vi "Power Law Fit with Offset.vi"(6 "method (LS)":T4 items=["Least Square", "Least Absolute Residual", "Bisquare"], 7 "Poisson Weight":bool, 8 "Error In":errorcluster, 9 "tolerance (1E-4)":dbl=0.0001 format="%#_3g", 10 "Weight (none)":dbl[](array[numeric]), 11 "Plot":T3) -> (0 "Error Out":errorcluster, 1 "Power Law with Baseline Fit":T3, 2 "Power Law Fit Results":T1, 3 "Power Law Fit":T3, 4 "Power Law + Baselien Fit Results":T1)   [LabVIEW 2021, in "AlliGator Camera Noise Influence on Lifetime.lvlib"]
uses:
  AlliGator Camera Noise Influence on Lifetime.lvlib
  Graphs/XY Graph/XY Graph Plot Data.ctl
  <vilib>/Analysis/6fits.llb/Curve Fitting Criteria.ctl
  Decay Fit Parameter Map/AlliGator Power Law Fit Results.ctl
  Power Law Parameters.ctl
  <userlib>/_OpenG.lib/array/array.llb/Filter 1D Array with Scalar (DBL)__ogtk.vi
  <userlib>/_OpenG.lib/array/array.llb/Delete Elements from 1D Array (DBL)__ogtk.vi
  <vilib>/Analysis/NI_AALPro.lvlib
  Error/Error.lvlib
  <userlib>/_OpenG.lib/array/array.llb/openg_array.lvlib
  Graphs/XY Graph/XY Graph Add-Ons.lvlib
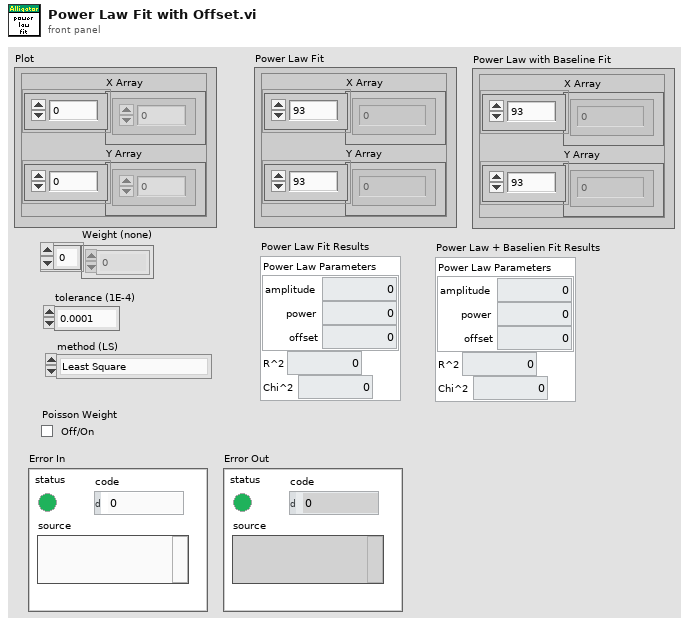
[diagram p1: front panel]
types:
  T1 = typedef "AlliGator Camera Noise Influence on Lifetime.lvlib/AlliGator Power Law Fit Results.ctl" = cluster{"Power Law Parameters":T2, "R^2":dbl, "Chi^2":dbl}
  T2 = typedef "AlliGator Camera Noise Influence on Lifetime.lvlib/Power Law Parameters.ctl" = cluster{"amplitude":dbl, "power":dbl, "offset":dbl}
  T3 = typedef "XY Graph Add-Ons.lvlib/XY Graph Plot Data.ctl" = cluster{"X Array":dbl[], "Y Array":dbl[]}
  T4 = typedef "NI_AALPro.lvlib/Curve Fitting Criteria.ctl" = u16
  T5 = cluster{"Power Law Parameters":T2, "R^2":dbl, "Chi^2":dbl}
  T6 = cluster{"amp min":dbl, "amp max":dbl, "power min":dbl, "power max":dbl, "offset min":dbl, "offset max":dbl}
  T7 = cluster{"amplitude":dbl, "power":dbl, "offset":dbl}
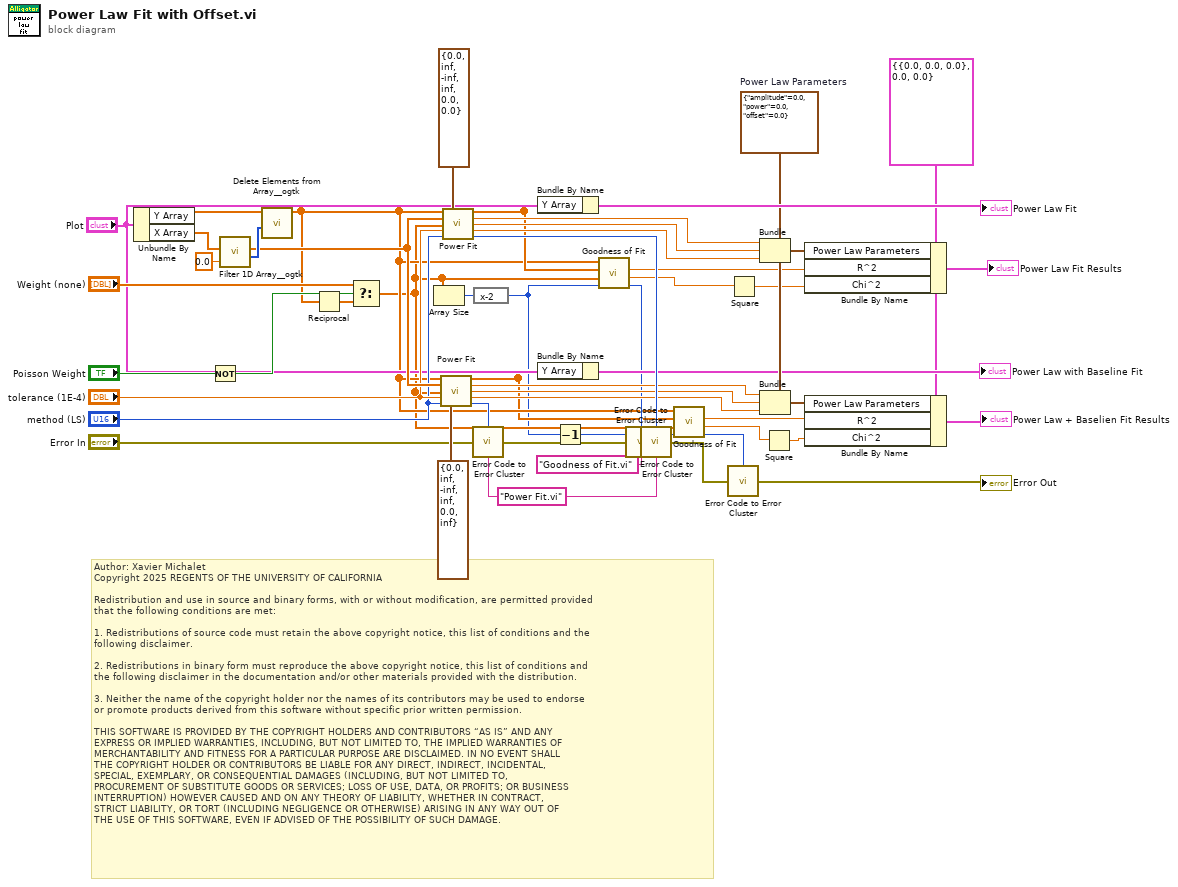
[diagram p0: block diagram]
diagram:
  w3 = T5 {"Power Law Parameters"={"amplitude"=0.0, "power"=0.0, "offset"=0.0}, "R^2"=0.0, "Chi^2"=0.0} ("Power Law + Baselien Fit Results")
  w32 = "Power Fit.vi" ("Error Source")
  w27 = T7 {"amplitude"=0.0, "power"=0.0, "offset"=0.0}  # Power Law Parameters
  # "Author: Xavier Michalet\nCopyright 2025 REGENTS OF THE UNIVERSITY OF CALIFORNIA\n\nRedistribution and use in source and binary forms, with or without modification, are permitted provided\nthat the following conditions are met:\n\n1. Redistributions of source code must retain the above copyright notice, this list of conditions and the\nfollowing disclaimer.\n\n2. Redistributions in binary form must reproduce the above copyright notice, this list of conditions and\nthe following disclaimer in the documentation and/or other materials provided with the distribution.\n\n3. Neither the name of the copyright holder nor the names of its contributors may be used to endorse \nor promote products derived from this software without specific prior written permission.\n\nTHIS SOFTWARE IS PROVIDED BY THE COPYRIGHT HOLDERS AND CONTRIBUTORS “AS IS” AND ANY \nEXPRESS OR IMPLIED WARRANTIES, INCLUDING, BUT NOT LIMITED TO, THE IMPLIED WARRANTIES OF\nMERCHANTABILITY AND FITNESS FOR A PARTICULAR PURPOSE ARE DISCLAIMED. IN NO EVENT SHALL\nTHE COPYRIGHT HOLDER OR CONTRIBUTORS BE LIABLE FOR ANY DIRECT, INDIRECT, INCIDENTAL, \nSPECIAL, EXEMPLARY, OR CONSEQUENTIAL DAMAGES (INCLUDING, BUT NOT LIMITED TO, \nPROCUREMENT OF SUBSTITUTE GOODS OR SERVICES; LOSS OF USE, DATA, OR PROFITS; OR BUSINESS\nINTERRUPTION) HOWEVER CAUSED AND ON ANY THEORY OF LIABILITY, WHETHER IN CONTRACT, \nSTRICT LIABILITY, OR TORT (INCLUDING NEGLIGENCE OR OTHERWISE) ARISING IN ANY WAY OUT OF\nTHE USE OF THIS SOFTWARE, EVEN IF ADVISED OF THE POSSIBILITY OF SUCH DAMAGE."
  n1 = Unbundle By Name("Plot") -> ("Y Array"=w47:dbl[], "X Array"=w46:dbl[])
  n2 = Not(x="Poisson Weight") -> (.not. x?=w41:bool)
  n3 = call-poly <userlib>:"Filter 1D Array__ogtk.vi"("items to filter"=0.0, "array"=w46) -> ("filtered item indices"=w44:i32[], "filtered array"=w38:dbl[])  [unwired: 4 in]
  n4 = call-poly <userlib>:"Delete Elements from Array__ogtk.vi"("indices"=w44, "array"=w47) -> ("array w/ subset deleted"=w15:dbl[])  [unwired: 8 in, 1 out]
  n5 = Reciprocal(x=w15) -> (1/x=w40:dbl[])
  n6 = Select(t="Weight (none)", s=w41, f=w40) -> (s? t:f=w13:dbl[])
  n7 = Array Size(array=w13) -> (size(s)=w24:i32)
  n8 = call <vilib>:"Power Fit.vi"("Y"=w15, "X"=w38, "Weight"=w13, "tolerance"="tolerance (1E-4)", "method"="method (LS)", "parameter bounds"=T6 {"amp min"=0.0, "amp max"=inf, "power min"=-inf, "power max"=inf, "offset min"=0.0, "offset max"=inf}) -> ("Best Power Fit"=w14:dbl[], "amplitude"=w30:dbl, "power"=w29:dbl, "offset"=w28:dbl, "error"=w34:i32)  [unwired: 4 in, 1 out]
  n9 = call <vilib>:"Power Fit.vi"("Y"=w15, "X"=w38, "Weight"=w13, "tolerance"="tolerance (1E-4)", "method"="method (LS)", "parameter bounds"=T6 {"amp min"=0.0, "amp max"=inf, "power min"=-inf, "power max"=inf, "offset min"=0.0, "offset max"=0.0}) -> ("Best Power Fit"=w25:dbl[], "amplitude"=w51:dbl, "power"=w50:dbl, "offset"=w49:dbl, "error"=w48:i32)  [unwired: 4 in, 1 out]
  n10 = call "Error Code to Error Cluster.vi"("Error Code"=w34, "Error Source"=w32, "Error In"="Error In") -> ("Error Out"=w22:errorcluster)  [unwired: 12 in]
  n11 = expression code="x-2"(w24) -> (w12:i32)
  n12 = Bundle By Name(cluster="Plot", "Y Array"=w25) -> (→"Power Law Fit":T3)
  n13 = Bundle By Name(cluster="Plot", "Y Array"=w14) -> (→"Power Law with Baseline Fit":T3)
  n14 = Decrement(x=w12) -> (x-1=w11:i32)
  n15 = call <vilib>:"Goodness of Fit.vi"("degree of freedom"=w12, "Weight"=w13, "Best Fit"=w25, "Y"=w15) -> ("error"=w23:i32, "RMSE"=w17:dbl, "R-square"=w18:dbl)  [unwired: 4 in, 1 out]
  n16 = call "Error Code to Error Cluster.vi"("Error Code"=w23, "Error Source"="Goodness of Fit.vi", "Error In"=w22) -> ("Error Out"=w21:errorcluster)  [unwired: 12 in]
  n17 = call "Error Code to Error Cluster.vi"("Error Code"=w48, "Error Source"=w32, "Error In"=w21) -> ("Error Out"=w9:errorcluster)  [unwired: 12 in]
  n18 = call <vilib>:"Goodness of Fit.vi"("degree of freedom"=w11, "Weight"=w13, "Best Fit"=w14, "Y"=w15) -> ("error"=w8:i32, "RMSE"=w5:dbl, "R-square"=w6:dbl)  [unwired: 4 in, 1 out]
  n19 = call "Error Code to Error Cluster.vi"("Error Code"=w8, "Error In"=w9) -> ("Error Out"=→"Error Out":errorcluster)  [unwired: 13 in]
  n20 = Square(x=w17) -> (x^2=w16:dbl)
  n21 = Bundle(cluster=w27, "amplitude"=w51, "power"=w50, "offset"=w49) -> (w19:T7)
  n22 = Bundle(cluster=w27, "amplitude"=w30, "power"=w29, "offset"=w28) -> (w10:T7)
  n23 = Square(x=w5) -> (x^2=w4:dbl)
  n24 = Bundle By Name(cluster=w3, "Power Law Parameters"=w19, "R^2"=w18, "Chi^2"=w16) -> (→"Power Law Fit Results":T5)
  n25 = Bundle By Name(cluster=w3, "Power Law Parameters"=w10, "R^2"=w6, "Chi^2"=w4) -> (→"Power Law + Baselien Fit Results":T5)
